vi "Remap arm encoder (SubVI).vi"(9 "encoder ticks per revolution":i32=4096, 10 "crossover to negative":i32=3072, 11 "Value":i32) -> (3 "Mapped":i32)   [LabVIEW 2019, in "Elevator.lvlib" / "Elevator Arm.lvclass"]
uses:
  Elevator Arm.lvclass
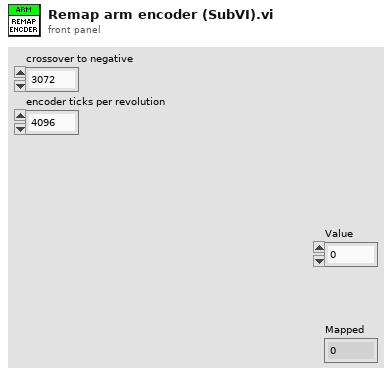
[diagram p1: front panel]
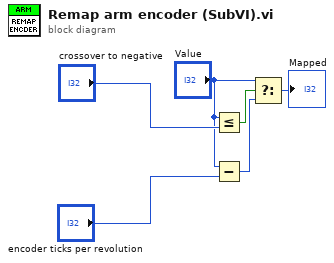
[diagram p0: block diagram]
diagram:
  n1 = Less Or Equal?(x="Value", y="crossover to negative") -> (x <= y?=w5:bool)
  n2 = Subtract(x="Value", y="encoder ticks per revolution") -> (x-y=w2:i32)
  n3 = Select(t="Value", s=w5, f=w2) -> (s? t:f=→"Mapped":i32)
